vi "NF87XX.reset attribute data.vi"(0 "i ref in":refnum<vi>, 5 "error in (no error)":errorcluster) -> (14 "i ref out":refnum<vi>, 19 "error out":errorcluster)   [LabVIEW 2014, in "NF87XX.lvlib"]
doc: "Resets the attribute data. This method should be executed in the constructor of THIS class.\n\nauthor: Dietrich Beck\ndata: 26-JUL-2004\n\n\nLicense Agreement for this software:\n\nCopyright (C)\nGesellschaft für Schwerionenforschung, GSI\nPlanckstr. 1\n64291 Darmstadt\nGermany\n\nContact: D.Beck@gsi.de \n\nThis program is free software; you can redistribute it and/or modify it under the terms of the GNU General Public License as published by the Free Software Foundation; either version 2 of the license, or (at your option) any later version.\n\nThis program is distributed in the hope that it will be useful, but WITHOUT ANY WARRANTY; without even the implied warranty of MERCHANTABILITY or FITNESS FOR A PARTICULAR PURPOSE. See the GNU General License for more details (http://www.gnu.org).\n\nGesellschaft für Schwerionenforschung, GSI\nPlanckstr. 1, 64291 Darmstadt, Germany\nFor all questions and ideas contact: M.Richter@gsi.de, H.Brand@gsi.de or D.Beck@gsi.de.\nLast update: 17-JUN-2004"
uses:
  NF87XX.lvlib
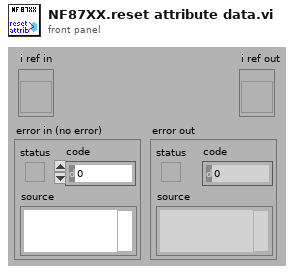
[diagram p1: front panel]
types:
  T1 = typedef "NF87XX.lvlib/NF87XX.i attribute.ctl" = cluster{"Con Settings":T2, "Drivers":T3[], "Status":cluster{"Service ID":i32, "Status":T6}, "Joystick available":bool, "VISA Resource":string}
  T2 = typedef "NewFocusPico - Driver np.lvlib/VISA & TCPIP Control.ctl" = cluster{"VISA or TCP/IP":bool, "Init Connection":bool, "Close Connection":bool, "Resource Name":refnum<visa-resource-name>, "hostname":string, "connection ID":refnum<k5>}
  T3 = typedef "NF87XX.lvlib/NF87XX.driver Settings.ctl" = cluster{"Name":string, "Driver Type":T4, "Pico Parameter type":T5, "Acceleration [Steps/s²]":cluster{"Motor 0":dbl, "Motor 1":dbl, "Motor 2":dbl}, "Start Velocity [Steps/s]":cluster{"Motor 0":dbl, "Motor 1":dbl, "Motor 2":dbl}, "Velocity [Steps/s]":cluster{"Motor 0":dbl, "Motor 1":dbl, "Motor 2":dbl}, "axis channel":i32, "Position":i32, "Position Service ID":i32}
  T4 = typedef "NF87XX.lvlib/NF87XX.driver Type.ctl" = enum16{"not defined", "3-ch open loop drv", "1-ch closed loop drv"}
  T5 = typedef "NewFocusPico - Driver np.lvlib/Pico Parameters.ctl" = cluster{"Pico Type":enum16{"Open-Loop Pico", "Close-Loop Pico", "Pico Ultra"}, "Acceleration (steps/sec^2)":string, "Velocity ( Hz)":string, "Driver":string, "Motor":string, "Channel":string, "Process Step":string}
  T6 = typedef "PH_StatusHandler.lvlib/PH_StatusHandler.Status.ctl" = i16
  T7 = cluster{"Motor 0":dbl, "Motor 1":dbl, "Motor 2":dbl}
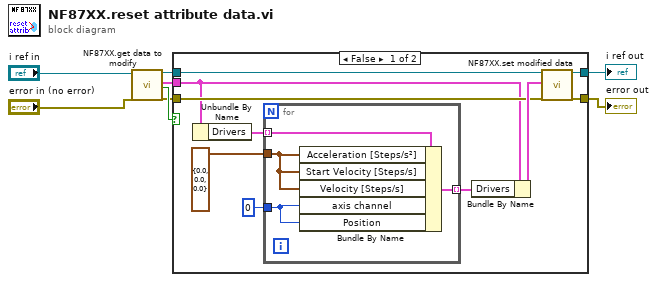
[diagram p0: block diagram]
diagram:
  n1 = call "NF87XX.get data to modify.vi"("i ref in"="i ref in", "error in (no error)"="error in (no error)") -> ("i ref out"=w7:refnum<vi>, "i attribute"=w6:T1, "timed out"=w8:bool, "error out"=w5:errorcluster)  [unwired: 14 in]
  n2 = case shown="False" w8 {
    tunnel: w7 -> [w18 w24]
    tunnel: w6 -> [w13 _]
    tunnel: [w14 w24] -> w1
    tunnel: [w15 w23] -> w2
    tunnel: w5 -> [w16 w23]
    frame False {
      n3 = Unbundle By Name(w13) -> ("Drivers"=w12:T3[])
      n4 = for {
        tunnel: w12 -> [w22] mode=indexing
        tunnel: T7 {"Motor 0"=0.0, "Motor 1"=0.0, "Motor 2"=0.0} ("Acceleration [Steps/s²]") -> [w21]
        tunnel: 0 ("axis channel") -> [w20]
        tunnel: [w19] -> w9 mode=indexing
        n5 = Bundle By Name(cluster=w22, "Acceleration [Steps/s²]"=w21, "Start Velocity [Steps/s]"=w21, "Velocity [Steps/s]"=w21, "axis channel"=w20, "Position"=w20) -> (w19:T3)
      }
      n6 = Bundle By Name(cluster=w13, "Drivers"=w9) -> (w17:T1)
      n7 = call "NF87XX.set modified data.vi"("i ref in"=w18, "i attribute"=w17, "error in (no error)"=w16) -> ("i ref out"=w14:refnum<vi>, "error out"=w15:errorcluster)  [unwired: 15 in]
    }
    frame True {
    }
  }
  "error out" <- w2
  "i ref out" <- w1
